vi "Plot Test.vi"() -> ()   [LabVIEW 2021]
uses:
  <vilib>/measure/NI_MABase.lvlib
panel:
  out "Cursor":refnum<vi>
  in  "sampling info 2":cluster{"Fs":dbl, "#s":dbl}={"Fs"=1000.0, "#s"=1000.0} {"Fs" format="%.2p"}
  out "Scope Screen":waveform(dbl)[](graph)
  in  "Cursor.Cursor Plot":i32
  in  "Active Y Scale":i32
  in  "Y Scale.Range:Minimum":dbl
  in  "Y Scale.Range:Maximum":dbl
  in  "sampling info":cluster{"Fs":dbl, "#s":dbl}={"Fs"=1000.0, "#s"=1000.0} {"Fs" format="%.2p"}
  in  "stop":bool
  in  "frequency 2":dbl=10.0 format="%0.2p"
  in  "amplitude 2":dbl=1.0 format="%0.2p"
  in  "amplitude":dbl=1.0 format="%0.2p"
  in  "frequency":dbl=10.0 format="%0.2p"
  # "Grid: 4th System color from left"
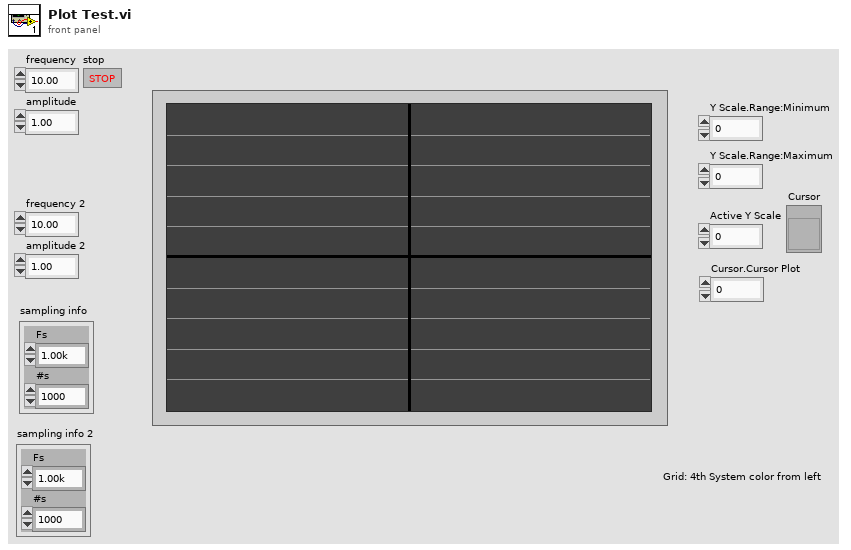
[diagram p1: front panel]
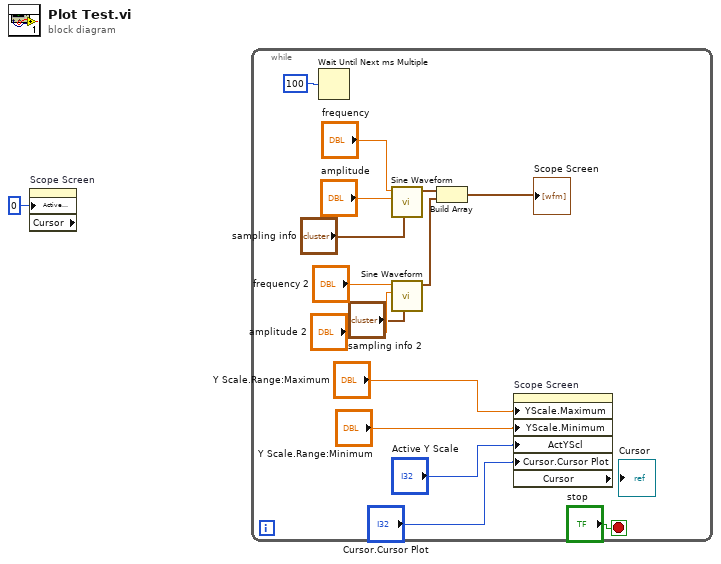
[diagram p0: block diagram]
diagram:
  n1 = property on="Scope Screen" class="WFGraph (strict)" props=["Active Cursor", "Cursor"]("Active Cursor"=u32 0) -> ()  [unwired: 2 in, 3 out]
  n2 = while {
    stop <- "stop" stop-if-true
    n3 = Wait Until Next ms Multiple(millisecond multiple=u32 100) -> ()  [unwired: 1 out]
    n4 = call <vilib>:"Sine Waveform.vi"("sampling info"="sampling info", "amplitude"="amplitude", "frequency"="frequency") -> ("signal out"=w10:waveform(dbl))  [unwired: 7 in, 1 out]
    n5 = call <vilib>:"Sine Waveform.vi"("sampling info"="sampling info 2", "amplitude"="amplitude 2", "frequency"="frequency 2") -> ("signal out"=w9:waveform(dbl))  [unwired: 7 in, 1 out]
    n6 = Build Array(w10, w9) -> (→"Scope Screen":waveform(dbl)[])
    n7 = property on="Scope Screen" class="WFGraph (strict)" props=["YScale", "Maximum", "YScale", "Minimum", "ActYScl", "Cursor", "Cursor Plot", "Cursor"]("YScale.Maximum"="Y Scale.Range:Maximum", "YScale.Minimum"="Y Scale.Range:Minimum", "ActYScl"="Active Y Scale", "Cursor.Cursor Plot"="Cursor.Cursor Plot") -> ()  [unwired: 2 in, 3 out]
  }
